vi "CalcIResponseArray.vi"(0 "Annular rings":cluster{"Radius":dbl, "a":dbl}[](array[cluster]) {"a" format="%.2f"; "Radius" format="%.2f"}, 1 "Pressure Calc":u16(ring)=1 items=["Pos Peak", "Neg peak", "Pk-Pk", "Steady State", "CW Drive", "Pii"], 2 "Full h(r,t)":bool, 5 "Variables in":T2={"Number of rings"=1, "sound spd (cm/s)"=150000, "z span (cm)"=4.0, "z steps"=20, "y span (cm)"=50.0, "y steps"=0, "time step (s)"=1e-08, "z"=0.0, "y"=0.0, "ref delay"=0.0, "freq (MHz)"=4.71, "cycles"=300} {"freq (MHz)" format="%.2f"; "z span (cm)" format="%.2f"; "y" format="%.2f"; "ref delay" format="%.2f"; "y span (cm)" format="%.2f"; "z" format="%.2f"; "time step (s)" format="%.2e"}, 7 "Calc":u16(ring) items=["One way", "RT Single Rings", "R/T Full Aperture"], 9 "Ring Number":i32, 11 "Waveform":dbl[](array[numeric]), 12 "Save Options":T1={"Save h Files?"=FALSE, "Save image data?"=FALSE, "Path"=path "E:/Test"}) -> (3 "delay pts":i32[](array[numeric]), 4 "h(r,t)":dbl[][](array[numeric]) format="%.2f", 15 "Y axis":dbl[](array[numeric]) format="%.2f")   [LabVIEW 2022 SP3]
panel:
  in  "Display 3-D?":bool
  in  "Index (row)":i32
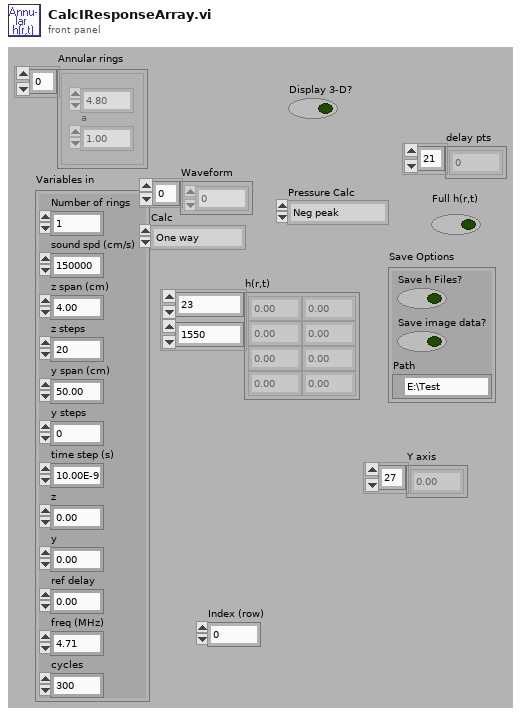
[diagram p1: front panel]
types:
  T1 = cluster{"Save h Files?":bool, "Save image data?":bool, "Path":path}
  T2 = cluster{"Number of rings":i32, "sound spd (cm/s)":i32, "z span (cm)":dbl, "z steps":i32, "y span (cm)":dbl, "y steps":i32, "time step (s)":sgl, "z":dbl, "y":dbl, "ref delay":dbl, "freq (MHz)":dbl, "cycles":i32}
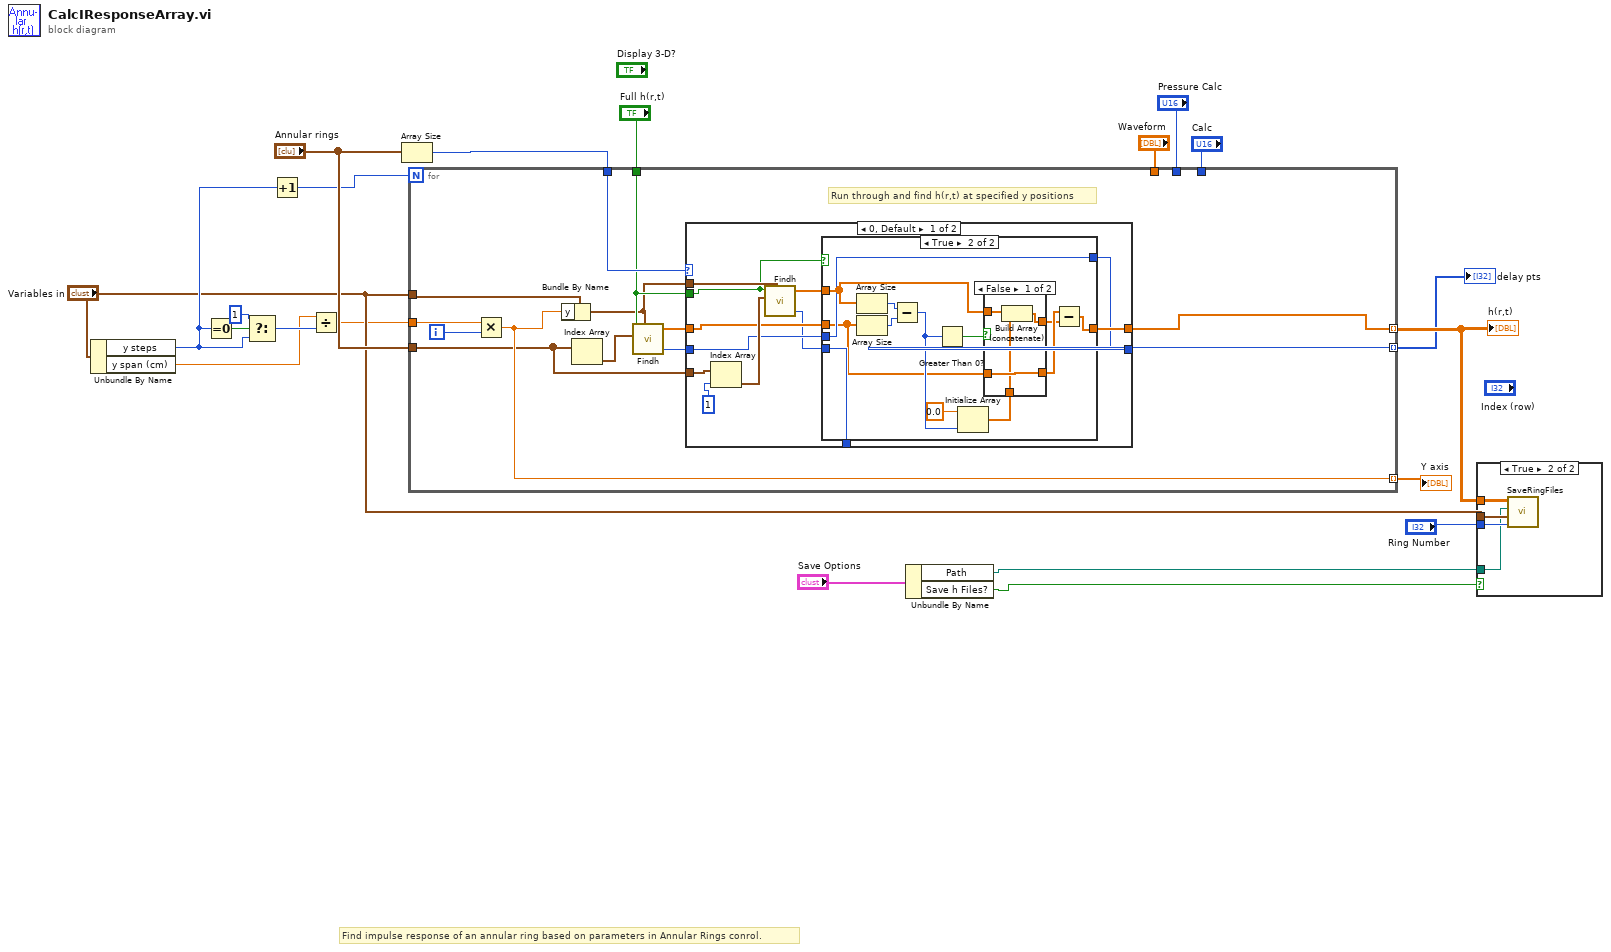
[diagram p0: block diagram]
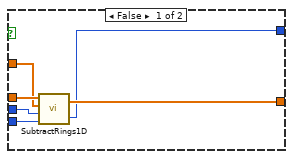
[diagram p3: hidden frame]
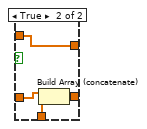
[diagram p4: hidden frame]
diagram:
  # "Find impulse response of an annular ring based on parameters in Annular Rings conrol."
  n1 = Unbundle By Name("Variables in") -> ("y steps"=w17:i32, "y span (cm)"=w15:dbl)
  n2 = Equal To 0?(x=w17) -> (x = 0?=w16:bool)
  n3 = Select(t=1, s=w16, f=w17) -> (s? t:f=w18:i32)
  n4 = Increment(x=w17) -> (x+1=w11:i32)
  n5 = Divide(x=w15, y=w18) -> (x/y=w13:dbl)
  n6 = Array Size(array="Annular rings") -> (size(s)=w7:i32)
  n7 = for {
    N: w11 -> [_]
    tunnel: [w22] -> w9 mode=indexing
    tunnel: "Variables in" -> [w34]
    tunnel: "Annular rings" -> [w30]
    tunnel: [w24] -> w8 mode=indexing
    tunnel: "Full h(r,t)" -> [w25]
    tunnel: w13 -> [w33]
    tunnel: [w31] -> w10 mode=indexing
    tunnel: w7 -> [w26]
    tunnel: "Calc" -> [_]
    tunnel: "Pressure Calc" -> [_]
    tunnel: "Waveform" -> [_]
    i -> [w32]
    # "Run through and find h(r,t) at specified y positions"
    n8 = Multiply(x=w33, y=w32) -> (x*y=w31:dbl)
    n9 = Bundle By Name(cluster=w34, "y"=w31) -> (w23:T2)
    n10 = Index Array(array=w30) -> (element=w29:cluster{"Radius":dbl, "a":dbl})  [unwired: 1 in]
    n11 = call "Findh.vi"("Full h(r,t)"=w25, "Trans Geometry"=w29, "Variables in"=w23) -> ("h(r,t)"=w28:dbl[], "delay pts"=w27:i32)  [unwired: 3 out]
    n12 = case shown="0, Default" w26 {
      tunnel: w23 -> [w45 _]
      tunnel: w30 -> [w44 _]
      tunnel: w25 -> [w41 _]
      tunnel: [w38 w73] -> w22
      tunnel: w28 -> [w40 w73]
      tunnel: [w37 w72] -> w24
      tunnel: w27 -> [w39 w72]
      tunnel: [w35 _] -> _
      frame 0, Default {
        n13 = Index Array(array=w44, index=1) -> (element=w42:cluster{"Radius":dbl, "a":dbl})
        n14 = call "Findh.vi"("Full h(r,t)"=w41, "Trans Geometry"=w42, "Variables in"=w45) -> ("h(r,t)"=w36:dbl[], "delay pts"=w35:i32)  [unwired: 3 out]
        n15 = case shown="True" w41 {
          tunnel: w40 -> [w48 w55]
          tunnel: w36 -> [w47 w56]
          tunnel: w35 -> [w51 _]
          tunnel: w39 -> [w46 w63]
          tunnel: [w50 w54] -> w38
          tunnel: [w49 w63] -> w37
          frame False {
            n16 = call "SubtractRings1D.vi"("delay pts inner"=w51, "delay pts outer"=w46, "h(r,t) ring inner"=w47, "h(r,t) ring outer"=w48) -> ("delay pts out"=w49:i32, "h(r,t) annulus"=w50:dbl[])
          }
          frame True {
            n17 = Array Size(array=w56) -> (size(s)=w57:i32)
            n18 = Array Size(array=w55) -> (size(s)=w58:i32)
            n19 = Subtract(x=w57, y=w58) -> (x-y=w60:i32)
            n20 = Greater Than 0?(x=w60) -> (x > 0?=w61:bool)
            n21 = Initialize Array(0.0, w60) -> (w62:dbl[])
            n22 = case shown="False" w61 {
              tunnel: w55 -> [w67 w71]
              tunnel: w62 -> [w64 w70]
              tunnel: [w67 w69] -> w53
              tunnel: w56 -> [w66 w68]
              tunnel: [w65 w68] -> w52
              frame False {
                n23 = Build Array (concatenate)(w66, w64) -> (w65:dbl[])
              }
              frame True {
                n24 = Build Array (concatenate)(w71, w70) -> (w69:dbl[])
              }
            }
            n25 = Subtract(x=w53, y=w52) -> (x-y=w54:dbl[])
          }
        }
      }
      frame 1 {
      }
    }
  }
  "h(r,t)" <- w9
  "Y axis" <- w10
  "delay pts" <- w8
  n26 = Unbundle By Name("Save Options") -> ("Path"=w5:path, "Save h Files?"=w4:bool)
  n27 = case shown="True" w4 {
    tunnel: "Ring Number" -> [_ w77]
    tunnel: w9 -> [_ w76]
    tunnel: "Variables in" -> [_ w75]
    tunnel: w5 -> [_ w74]
    frame False {
    }
    frame True {
      n28 = call "SaveRingFiles.vi"("h(r,t)"=w76, "Path"=w74, "Variables in"=w75, "Ring Number"=w77) -> ()  [unwired: 1 in, 4 out]
    }
  }
